vi "Do.vi"(8 "error in (no error)":errorcluster, 10 "Actor in":refnum<class "Actor.lvclass">, 11 "Right Click Menu Activated Msg in":refnum<class "Right Click Menu Activated Msg.lvclass">) -> (0 "error out":errorcluster, 2 "Actor out":refnum<class "Actor.lvclass">)   [LabVIEW 2020, in "SubPanel User Interface.lvlib" / "Right Click Menu Activated Msg.lvclass"]
doc: "This VI delivers the message to the actor by calling the appropriate method(s) on the actor."
uses:
  Right Click Menu Activated Msg.lvclass
  <vilib>/ActorFramework/Actor/Actor.lvclass
  SubPanel User Interface/SubPanel User Interface.lvclass
  C:/Program Files/National Instruments/LabVIEW 2020/vi.lib/ActorFramework/Actor/Actor.lvclass
  Right Click Menu Activated Msg.lvclass/Right Click Menu Activated Msg.ctl
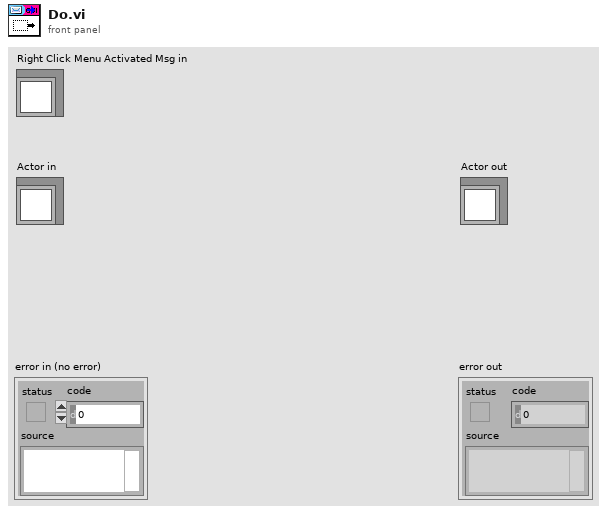
[diagram p1: front panel]
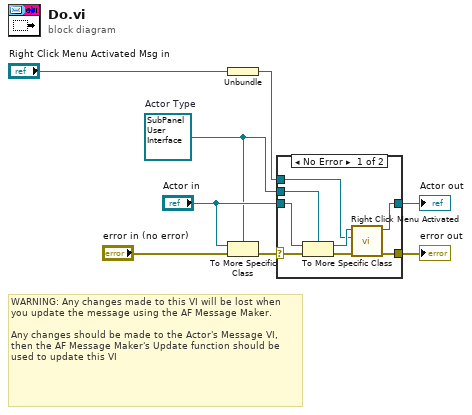
[diagram p0: block diagram]
diagram:
  w3 = refnum<class "SubPanel User Interface.lvclass"> refnum  # Actor Type
  # "WARNING: Any changes made to this VI will be lost when you update the message using the AF Message Maker.\n\nAny changes should be made to the Actor's Message VI, then the AF Message Maker's Update function should be used to update this VI"
  n1 = Unbundle("Right Click Menu Activated Msg in") -> (w2:refnum<k9>)
  n2 = To More Specific Class(target class=w3, reference="Actor in", error in="error in (no error)") -> (error out=w7:errorcluster)  [unwired: 1 out]
  n3 = case shown="No Error" w7 {
    selector: w7 -> [w16 w18]
    tunnel: [w11 w18] -> w6
    tunnel: [w10 w17] -> w5
    tunnel: "Actor in" -> [w15 w17]
    tunnel: w3 -> [w14 _]
    tunnel: w2 -> [w9 _]
    frame No Error {
      n4 = To More Specific Class ("Actor Cast")(target class=w14, reference=w15, error in=w16) -> (specific class reference=w13:refnum<class "SubPanel User Interface.lvclass">, error out=w12:errorcluster)
      n5 = call "Right Click Menu Activated.vi"("error in (no error)"=w12, "MenuRef"=w9, "SubPanel User Interface in"=w13) -> ("error out"=w11:errorcluster, "SubPanel User Interface out"=w10:refnum<class "SubPanel User Interface.lvclass">)  [unwired: 7 in]
    }
    frame Error {
    }
  }
  "error out" <- w6
  "Actor out" <- w5
